vi "GOOPUtil_EatError.vi"(3 "error in":errorcluster) -> ()   [LabVIEW 2020, in "GOOPUtility.lvlib"]
doc: "Eats the error.\nNom nom"
uses:
  <vilib>/addons/GOOPUtility/GOOPUtility.lvlib
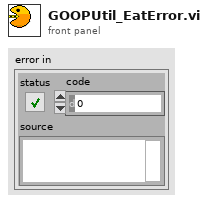
[diagram p1: front panel]
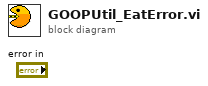
[diagram p0: block diagram]
diagram:
